vi "CMD_LOADCONFIG.vi"(6 "Gantry in":refnum<class "Gantry.lvclass">, 8 "error in (no error)":errorcluster, 10 "Arguments":string[](array[string]), 11 "gScript Interpreter in":refnum<class "gScript Interpreter.lvclass">) -> (0 "error out":errorcluster, 3 "gScript Interpreter out":refnum<class "gScript Interpreter.lvclass">, 4 "Gantry out":refnum<class "Gantry.lvclass">)   [LabVIEW 2024, in "gScript Interpreter.lvclass"]
uses:
  gScript Interpreter.lvclass
  Shared Components/Gantry Class/Gantry.lvclass
  Shared Components/FlexWorktable/FlexWorktable.lvclass
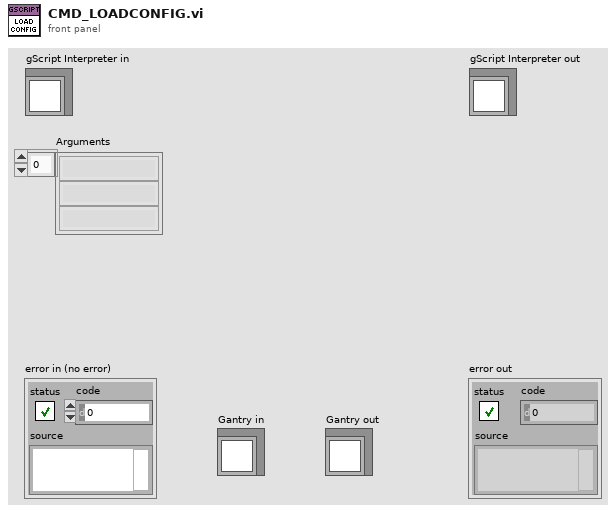
[diagram p1: front panel]
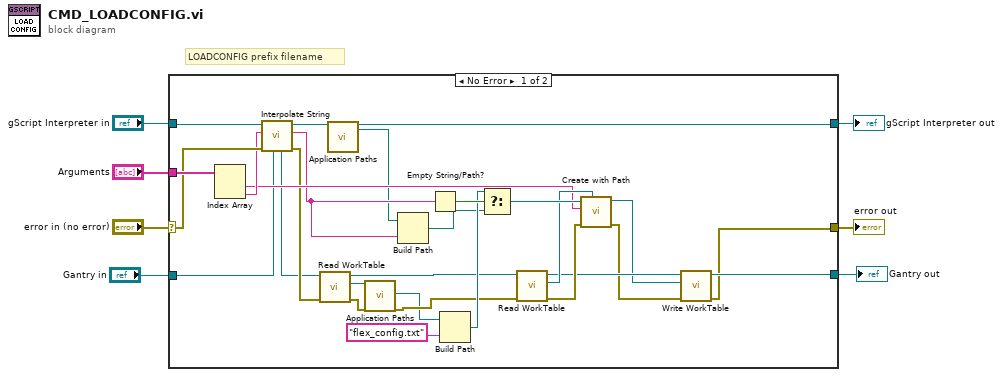
[diagram p0: block diagram]
diagram:
  # "LOADCONFIG prefix filename"
  n1 = case shown="No Error" "error in (no error)" {
    selector: "error in (no error)" -> [w34 w39]
    tunnel: [w21 w39] -> w6
    tunnel: [w16 w38] -> w4
    tunnel: "gScript Interpreter in" -> [w35 w38]
    tunnel: "Arguments" -> [w36 _]
    tunnel: "Gantry in" -> [w9 w37]
    tunnel: [w22 w37] -> w1
    frame No Error {
      n2 = Index Array(array=w36) -> (element #1=w27:string, element #2=w33:string)  [unwired: 2 in]
      n3 = call-dynamic "Interpolate String.vi"("Gantry in"=w9, "error in (no error)"=w34, "Input String"=w33, "gScript Interpreter in"=w35) -> ("error out"=w14:errorcluster, "Output String"=w19:string, "gScript Interpreter out"=w18:refnum<class "gScript Interpreter.lvclass">, "Gantry out"=w8:refnum<class "Gantry.lvclass">)  [unwired: 4 in]
      n4 = call-dynamic "Read WorkTable.vi"("error in"=w14, "Gantry Class in"=w8) -> ("error out"=w12:errorcluster, "Worktable"=w13:refnum<class "FlexWorktable.lvclass">, "Gantry Class out"=w15:refnum<class "Gantry.lvclass">)  [unwired: 7 in]
      n5 = call "Application Paths.vi"("gScript Interpreter in"=w18) -> ("gScript Interpreter out"=w16:refnum<class "gScript Interpreter.lvclass">, "Project Path"=w17:path)  [unwired: 13 in, 4 out]
      n6 = call "Application Paths.vi"("FlexWorktable in"=w13, "error in (no error)"=w12) -> ("Config Path"=w10:path, "error out"=w11:errorcluster)  [unwired: 11 in, 5 out]
      n7 = Build Path(base path=w17, name or relative path=w19) -> (appended path=w20:path)
      n8 = Empty String/Path?(string/path=w19) -> (empty?=w31:bool)
      n9 = Build Path(base path=w10, name or relative path="flex_config.txt") -> (appended path=w30:path)
      n10 = Select(t=w30, s=w31, f=w20) -> (s? t:f=w29:path)
      n11 = call-dynamic "Read WorkTable.vi"("error in"=w11, "Gantry Class in"=w15) -> ("error out"=w26:errorcluster, "Worktable"=w28:refnum<class "FlexWorktable.lvclass">, "Gantry Class out"=w25:refnum<class "Gantry.lvclass">)  [unwired: 7 in]
      n12 = call "Create with Path.vi"("Existing FlexWorktable"=w28, "error in (no error)"=w26, "prefix"=w27, "flex_config path"=w29) -> ("error out"=w23:errorcluster, "FlexWorktable out"=w24:refnum<class "FlexWorktable.lvclass">)  [unwired: 6 in]
      n13 = call-dynamic "Write WorkTable.vi"("error in (no error)"=w23, "FlexWorktable"=w24, "Gantry Class in"=w25) -> ("error out"=w21:errorcluster, "Gantry Class out"=w22:refnum<class "Gantry.lvclass">)  [unwired: 7 in]
    }
    frame Error {
    }
  }
  "error out" <- w6
  "gScript Interpreter out" <- w4
  "Gantry out" <- w1
